vi "CreateCurveNamesvb1.vi"(8 "error in":errorcluster, 9 "NomDon":string[](array[string])=["RTêta;", "X&Y;"], 10 "IndCourbe":i64 caption="Numéro de Balayage", 11 "Experiment.lvclass In":refnum<class "Experiment.lvclass">) -> (0 "error out":errorcluster, 1 "VarPar list":string[](array[string]), 2 "Scan list":string[](array[string]), 3 "Experiment.lvclass Out":refnum<class "Experiment.lvclass">, 4 "ScanTableSize":i32[](array[numeric]))   [LabVIEW 2012]
doc: "Ce Vi créer la ligne d'entête du fichier texte de sauvegarde à partir du nombre de courbe voulu."
uses:
  DevicesClass/BaseDevice/BaseDevice.lvclass
  Calculations Class/Calculations.lvclass
  Experiment.lvclass
panel:
  out "DataQIndex":cluster{"Tableau":i32[]}[](array[cluster])
  out "CalcQIndex":cluster{"Tableau":i32[]}[](array[cluster])
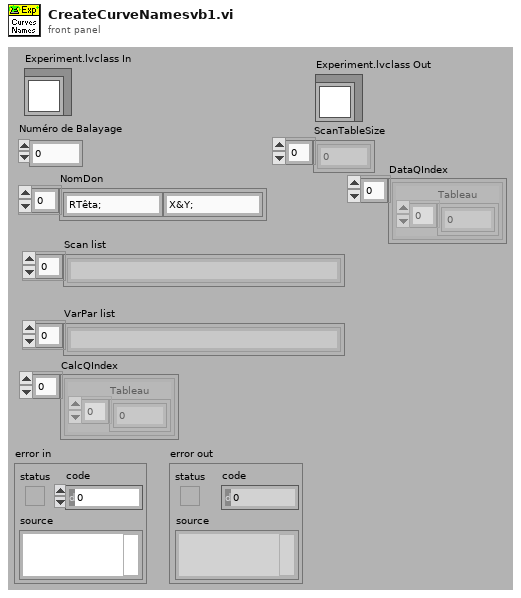
[diagram p1: front panel]
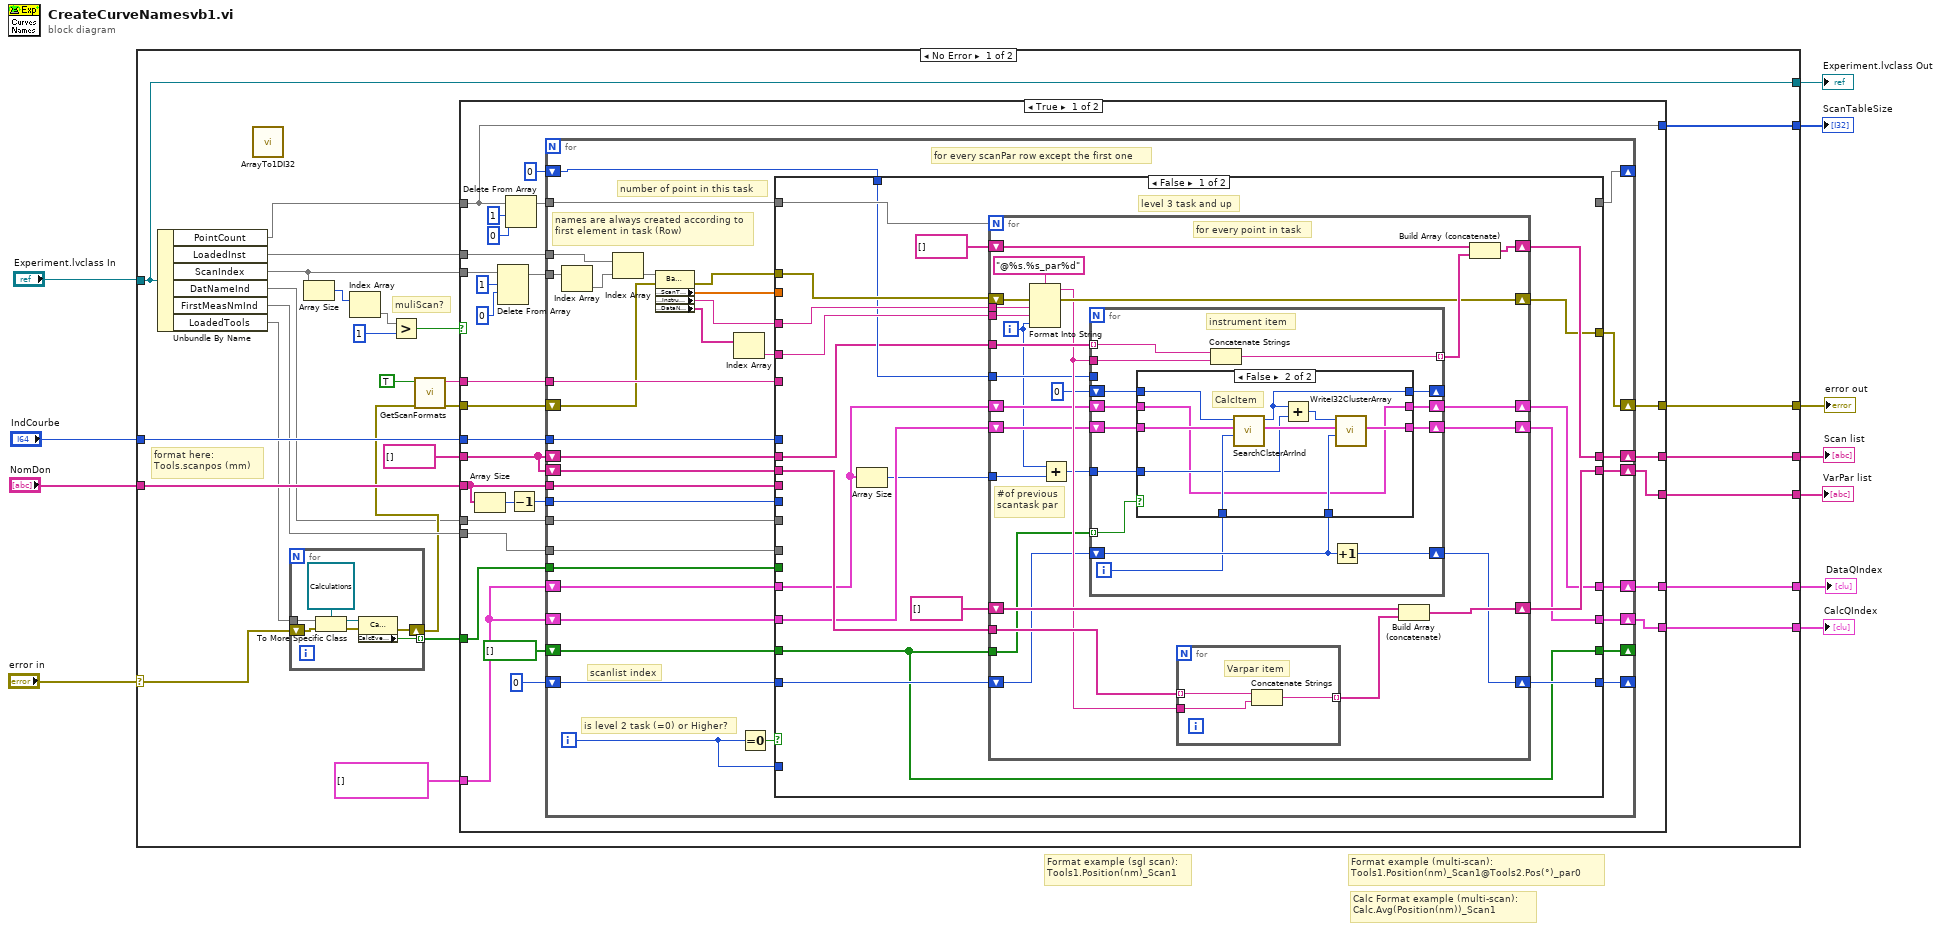
[diagram p0: block diagram]
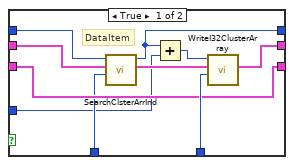
[diagram p2: hidden frame]
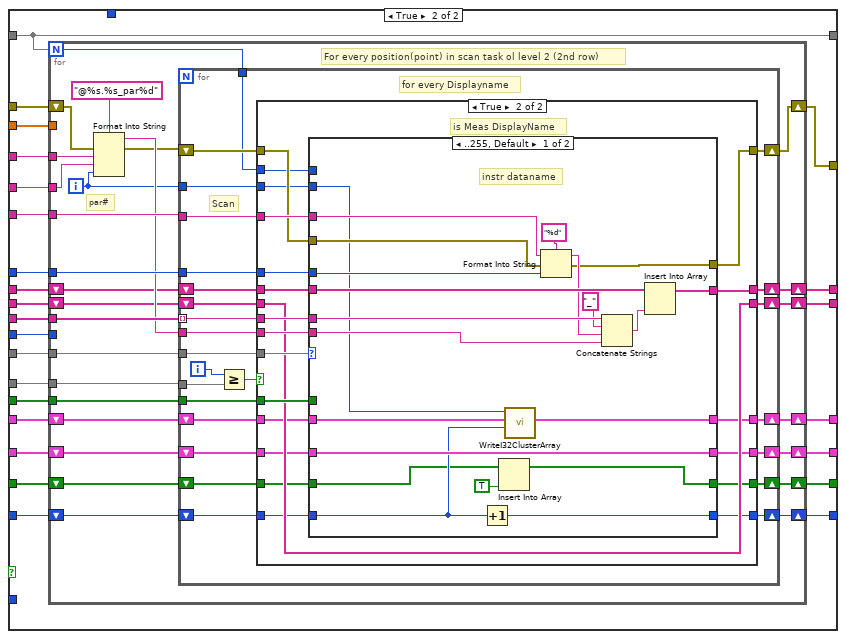
[diagram p3: hidden frame]
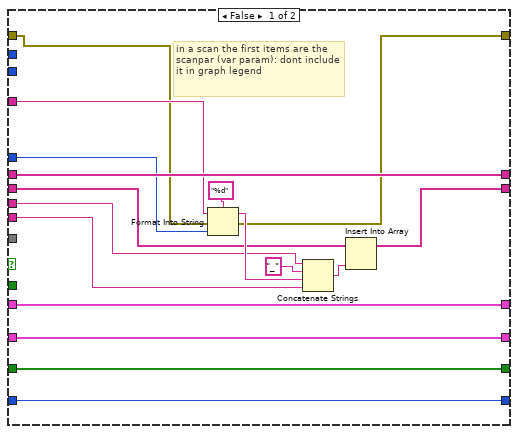
[diagram p4: hidden frame]
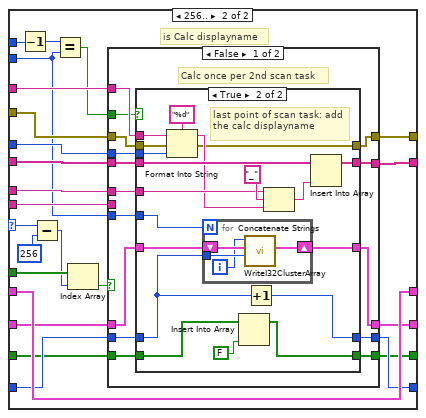
[diagram p5: hidden frame]
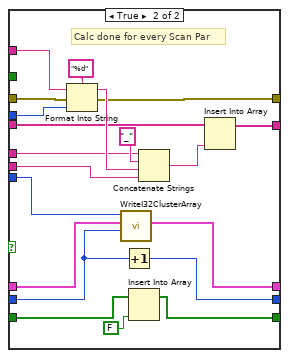
[diagram p7: hidden frame]
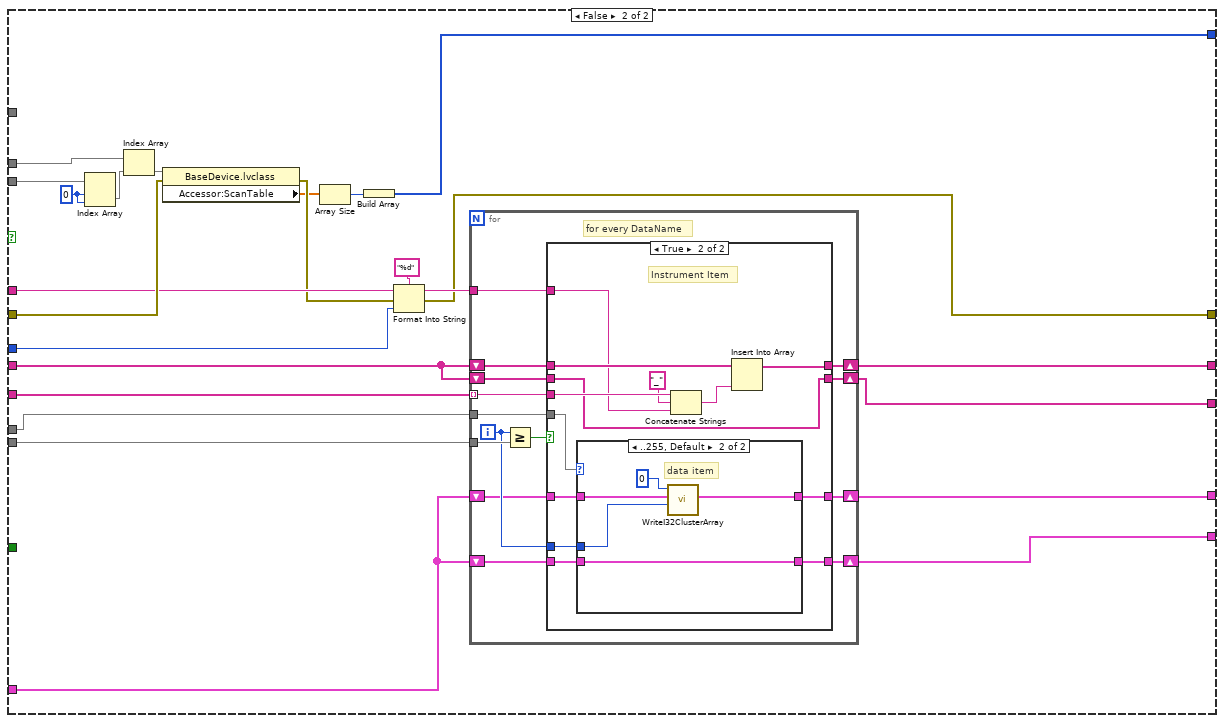
[diagram p8: hidden frame]
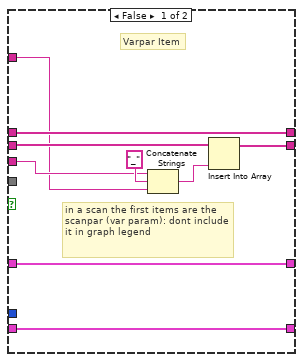
[diagram p9: hidden frame]
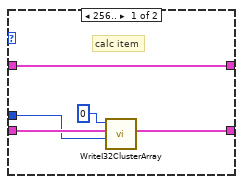
[diagram p10: hidden frame]
diagram:
  # "Calc Format example (multi-scan):\nCalc.Avg(Position(nm))_Scan1"
  # "Format example (multi-scan):\nTools1.Position(nm)_Scan1@Tools2.Pos(°)_par0"
  # "Format example (sgl scan):\nTools1.Position(nm)_Scan1"
  n1 = case shown="No Error" "error in" {
    selector: "error in" -> [w21 w486]
    tunnel: [w29 w486] -> w10
    tunnel: [w34 _] -> w9
    tunnel: "NomDon" -> [w35 _]
    tunnel: "Experiment.lvclass In" -> [w18 w485]
    tunnel: "IndCourbe" -> [w37 _]
    tunnel: [w18 w485] -> w5
    tunnel: [w26 _] -> w4
    tunnel: [w17 _] -> w3
    tunnel: [w14 _] -> w2
    tunnel: [w13 _] -> w1
    frame No Error {
      # "format here:\nTools.scanpos (mm)"
      # "muliScan?"
      n2 = Unbundle By Name(w18) -> ("PointCount"=w23, "LoadedInst"=w30, "ScanIndex"=w31, "DatNameInd"=w16, "FirstMeasNmInd"=w28, "LoadedTools"=w22)
      n3 = call <userlib>:"ArrayTo1DI32.vi"() -> ()  [unwired: 9 in, 3 out]
      n4 = for {
        tunnel: w22 -> [w42]
        shift-right: [w40] -> w20
        shift-left: w21 -> [w41]
        tunnel: [w39] -> w19 mode=indexing
        n5 = To More Specific Class(target class=refnum<class "Calculations.lvclass"> refnum ("Calculations.lvclass"), reference=w42, error in=w41) -> (specific class reference=w44:refnum<class "Calculations.lvclass">, error out=w45:errorcluster)
        n6 = property class="Calculations.lvclass"(reference=w44, error in=w45) -> (error out=w40:errorcluster, "CalcEveryScanPar"=w39:bool)  [unwired: 1 out]
      }
      n7 = Array Size(array=w31) -> (size(s)=w25:i32)
      n8 = Index Array(array=w25) -> (element=w24)  [unwired: 1 in]
      n9 = Greater?(x=w24, y=1) -> (0:w27:bool)
      n10 = call "GetScanFormats.vi"("ErrorIn(No Error)"=w20, "Scan(T)"=TRUE) -> ("sortie d'erreur"=w36:errorcluster, "Prefixe"=w38:string)  [unwired: 7 in, 1 out]
      n11 = case shown="True" w27 {
        tunnel: w38 -> [w73 w427]
        tunnel: w37 -> [w72 w428]
        tunnel: w36 -> [w71 w432]
        tunnel: w35 -> [w58 w438]
        tunnel: [w66 w437] -> w34
        tunnel: string[] [] -> [w53 w431]
        tunnel: w31 -> [w70 w435]
        tunnel: w30 -> [w69 w434]
        tunnel: [w68 w420] -> w29
        tunnel: w28 -> [w67 w436]
        tunnel: [w54 w433] -> w26
        tunnel: w23 -> [w54 _]
        tunnel: w16 -> [w59 w424]
        tunnel: w19 -> [w55 _]
        tunnel: [w52 w430] -> w17
        tunnel: cluster{"Tableau":i32[]}[] [] ("CalcQIndex") -> [w50 w422]
        tunnel: [w49 w421] -> w14
        tunnel: [w48 w423] -> w13
        frame True {
          n12 = Array Size(array=w58) -> (size(s)=w57:i32)
          n13 = Delete From Array(array=w70, length=1 ("longueur"), index (row)=0 ("indice (ligne)")) -> (array with subset deleted=w65)  [unwired: 1 in, 1 out]
          n14 = Delete From Array(array=w54, length=1 ("longueur"), index=0 ("indice")) -> (array with subset deleted=w61)  [unwired: 1 out]
          n15 = Decrement(x=w57) -> (x-1=w56:i32)
          n16 = for {
            tunnel: w73 -> [w108]
            tunnel: w72 -> [w107]
            tunnel: w58 -> [w106]
            tunnel: w65 -> [w105]
            tunnel: w69 -> [w104]
            shift-right: [w102] -> w68
            shift-left: w71 -> [w103]
            tunnel: w67 -> [w101]
            shift-right: [w98] -> w66
            shift-left: w53 -> [w97]
            tunnel: w61 -> [w78]
            tunnel: w59 -> [w90]
            tunnel: w55 -> [w89]
            tunnel: w56 -> [w88]
            shift-right: [w85] -> w52
            shift-left: w53 -> [w86]
            shift-right: [w83] -> _
            shift-left: 0 ("Numérique") -> [w84]
            shift-right: [w79] -> w49
            shift-left: w50 -> [w80]
            shift-right: [w81] -> w48
            shift-left: w50 -> [w82]
            shift-right: [w77] -> _
            shift-left: 0 ("Numérique") -> [w76]
            shift-right: [w74] -> _
            shift-left: bool[] [] -> [w75]
            i -> [w87]
            # "scanlist index"
            # "is level 2 task (=0) or Higher?"
            # "number of point in this task"
            # "names are always created according to first element in task (Row)"
            # "for every scanPar row except the first one"
            n17 = Index Array(array=w105) -> (element=w95)  [unwired: 1 in]
            n18 = Index Array(array=w104, index=w95) -> (element=w94)
            n19 = property class="BaseDevice.lvclass"(reference=w94, error in=w103) -> (error out=w96:errorcluster, "Accessor:ScanTable"=w92:dbl[], "Accessor:InstrumentName"=w99:string, "Accessor:DataNames"=w93:string[])  [unwired: 1 out]
            n20 = Index Array(array=w93) -> (element=w100:string)  [unwired: 1 in]
            n21 = Equal To 0?(x=w87) -> (x = 0?=w91:bool)
            n22 = case shown="False" w91 {
              tunnel: w108 -> [_ w216]
              tunnel: w107 -> [_ w215]
              tunnel: w106 -> [_ w214]
              tunnel: [w126 w213] -> w102
              tunnel: w101 -> [_ w212]
              tunnel: w100 -> [w124 w211]
              tunnel: w99 -> [w123 w210]
              tunnel: [w127 w209] -> w98
              tunnel: w97 -> [w113 w208]
              tunnel: w78 -> [w125 w194]
              tunnel: w96 -> [w128 w207]
              tunnel: w92 -> [_ w206]
              tunnel: w90 -> [_ w205]
              tunnel: w89 -> [_ w204]
              tunnel: w88 -> [_ w203]
              tunnel: w87 -> [_ _]
              tunnel: w86 -> [w122 w202]
              tunnel: [w121 w201] -> w85
              tunnel: w84 -> [w119 w200]
              tunnel: [w118 w199] -> w83
              tunnel: w82 -> [w112 w198]
              tunnel: [w115 w197] -> w81
              tunnel: w80 -> [w120 w196]
              tunnel: [w114 w195] -> w79
              tunnel: [_ w194] -> w77
              tunnel: w76 -> [w117 _]
              tunnel: w75 -> [w116 w193]
              tunnel: [w116 w192] -> w74
              frame False {
                # "level 3 task and up"
                n23 = Array Size(array=w112) -> (size(s)=w111:i32)
                n24 = for {
                  N: w125 -> [_]
                  tunnel: w123 -> [w154]
                  tunnel: w124 -> [w153]
                  shift-right: [w149] -> w126
                  shift-left: w128 -> [w152]
                  tunnel: w113 -> [w151]
                  shift-right: [w148] -> w127
                  shift-left: string[] [] -> [w147]
                  shift-right: [w145] -> w121
                  shift-left: string[] [] -> [w144]
                  tunnel: w122 -> [w143]
                  shift-right: [w133] -> w114
                  shift-left: w120 -> [w135]
                  shift-right: [w132] -> w118
                  shift-left: w119 -> [w140]
                  shift-right: [w134] -> w115
                  shift-left: w112 -> [w137]
                  tunnel: w117 -> [w139]
                  tunnel: w116 -> [w138]
                  tunnel: w111 -> [w131]
                  i -> [w130]
                  # "#of previous\nscantask par"
                  # "for every point in task"
                  n25 = Format Into String(format string="@%s.%s_par%d" ("chaîne de format"), error in=w152, w154, w153, w130) -> (resulting string=w141:string, error out=w149:errorcluster)  [unwired: 1 in]
                  n26 = Add(x=w130, y=w131) -> (x+y=w129:i32)
                  n27 = for {
                    tunnel: w151 -> [w168] mode=indexing
                    tunnel: [w167] -> w150 mode=indexing
                    tunnel: w141 -> [w166]
                    tunnel: w139 -> [_]
                    tunnel: w138 -> [w165] mode=indexing
                    shift-right: [w162] -> w134
                    shift-left: w137 -> [w164]
                    shift-right: [w156] -> _
                    shift-left: 0 -> [w157]
                    shift-right: [w160] -> w133
                    shift-left: w135 -> [w161]
                    shift-right: [w159] -> w132
                    shift-left: w140 -> [w163]
                    tunnel: w129 -> [w155]
                    i -> [w158]
                    # "instrument item"
                    n28 = case shown="False" w165 {
                      tunnel: w164 -> [w175 w179]
                      tunnel: w163 -> [w178 w188]
                      tunnel: [w177 w179] -> w162
                      tunnel: w161 -> [w176 w181]
                      tunnel: [w176 w180] -> w160
                      tunnel: w158 -> [w173 w186]
                      tunnel: w157 -> [w172 w185]
                      tunnel: [w171 w184] -> w156
                      tunnel: w155 -> [w170 w183]
                      frame True {
                        # "DataItem"
                        n29 = call "SearchClsterArrInd.vi"("SearchData"=w173, "array"=w175, "ClusterInd"=w172) -> ("output array"=w174:cluster{"Tableau":i32[]}[], "ClusterInd Out"=w171:i32)  [unwired: 6 in, 1 out]
                        n30 = Add(x=w171, y=w170) -> (x+y=w169:i32)
                        n31 = call <userlib>:"WriteI32ClusterArray.vi"("Data"=w178, "array"=w174, "ClusterInd"=w169) -> ("output array"=w177:cluster{"Tableau":i32[]}[])  [unwired: 7 in, 1 out]
                      }
                      frame False {
                        # "CalcItem"
                        n32 = call "SearchClsterArrInd.vi"("SearchData"=w186, "array"=w181, "ClusterInd"=w185) -> ("output array"=w187:cluster{"Tableau":i32[]}[], "ClusterInd Out"=w184:i32)  [unwired: 6 in, 1 out]
                        n33 = Add(x=w184, y=w183) -> (x+y=w182:i32)
                        n34 = call <userlib>:"WriteI32ClusterArray.vi"("Data"=w188, "array"=w187, "ClusterInd"=w182) -> ("output array"=w180:cluster{"Tableau":i32[]}[])  [unwired: 7 in, 1 out]
                      }
                    }
                    n35 = Concatenate Strings(w168, w166) -> (w167:string)
                    n36 = Increment(x=w163) -> (x+1=w159:i32)
                  }
                  n37 = for {
                    tunnel: w143 -> [w191] mode=indexing
                    tunnel: [w190] -> w146 mode=indexing
                    tunnel: w141 -> [w189]
                    # "Varpar item"
                    n38 = Concatenate Strings(w191, w189) -> (w190:string)
                  }
                  n39 = Build Array (concatenate)(w144, w146) -> (w145:string[])
                  n40 = Build Array (concatenate)(w147, w150) -> (w148:string[])
                }
              }
              frame True {
                n41 = for {
                  N: w194 -> [w230]
                  tunnel: w216 -> [w243]
                  tunnel: w215 -> [w242]
                  tunnel: w214 -> [w241]
                  shift-right: [w227] -> w213
                  shift-left: w207 -> [w239]
                  tunnel: w212 -> [w240]
                  tunnel: w211 -> [w238]
                  tunnel: w210 -> [w237]
                  shift-right: [w228] -> w209
                  shift-left: w208 -> [w235]
                  tunnel: w206 -> [_]
                  tunnel: w205 -> [w232]
                  tunnel: w204 -> [w231]
                  tunnel: w203 -> [_]
                  shift-right: [w225] -> w201
                  shift-left: w202 -> [w226]
                  shift-right: [w223] -> w199
                  shift-left: w200 -> [w224]
                  shift-right: [w221] -> w197
                  shift-left: w198 -> [w222]
                  shift-right: [w219] -> w195
                  shift-left: w196 -> [w220]
                  shift-right: [w217] -> w192
                  shift-left: w193 -> [w218]
                  i -> [w229]
                  # "par#"
                  # "For every position(point) in scan task ol level 2 (2nd row)"
                  n42 = Format Into String(format string="@%s.%s_par%d" ("chaîne de format"), error in=w239, w237, w238, w229) -> (resulting string=w236:string, error out=w234:errorcluster)  [unwired: 1 in]
                  n43 = for {
                    tunnel: w243 -> [w263]
                    tunnel: w241 -> [w266] mode=indexing
                    shift-right: [w267] -> w228
                    shift-left: w235 -> [w268]
                    tunnel: w242 -> [w264]
                    shift-right: [w254] -> w227
                    shift-left: w234 -> [w262]
                    tunnel: w240 -> [w261]
                    tunnel: w236 -> [w260]
                    tunnel: w232 -> [w259]
                    tunnel: w231 -> [w258]
                    tunnel: w230 -> [w256]
                    tunnel: w229 -> [w255]
                    shift-right: [w252] -> w225
                    shift-left: w226 -> [w253]
                    shift-right: [w250] -> w223
                    shift-left: w224 -> [w251]
                    shift-right: [w248] -> w221
                    shift-left: w222 -> [w249]
                    shift-right: [w246] -> w219
                    shift-left: w220 -> [w247]
                    shift-right: [w245] -> w217
                    shift-left: w218 -> [w244]
                    i -> [w257]
                    # "Scan"
                    # "for every Displayname"
                    n44 = Greater Or Equal?(x=w257, y=w261) -> (x >= y?=w265:bool)
                    n45 = case shown="True" w265 {
                      tunnel: w268 -> [w285 w306]
                      tunnel: [w285 w305] -> w267
                      tunnel: w266 -> [w279 w304]
                      tunnel: w264 -> [w273 w300]
                      tunnel: w263 -> [w280 w303]
                      tunnel: w262 -> [w277 w302]
                      tunnel: w260 -> [w278 w301]
                      tunnel: w259 -> [_ w298]
                      tunnel: w258 -> [_ w299]
                      tunnel: w256 -> [_ w297]
                      tunnel: w255 -> [_ w296]
                      tunnel: [w276 w295] -> w254
                      tunnel: w253 -> [w275 w294]
                      tunnel: [w274 w294] -> w252
                      tunnel: w251 -> [w272 w289]
                      tunnel: [w272 w288] -> w250
                      tunnel: w249 -> [w271 w293]
                      tunnel: [w271 w292] -> w248
                      tunnel: w247 -> [w270 w291]
                      tunnel: [w270 w290] -> w246
                      tunnel: [w269 w286] -> w245
                      tunnel: w244 -> [w269 w287]
                      frame False {
                        # "in a scan the first items are the scanpar (var param): dont include it in graph legend"
                        n46 = Format Into String(format string="%d" ("chaîne de format"), initial string=w280, error in=w277, w273) -> (resulting string=w283:string, error out=w276:errorcluster)
                        n47 = Concatenate Strings(w279, "_" ("chaîne"), w283, w278) -> (w284:string)
                        n48 = Insert Into Array(array=w275, new element=w284) -> (w274:string[])  [unwired: 1 in]
                      }
                      frame True {
                        # "is Meas DisplayName"
                        n49 = case shown="..255, Default" w298 {
                          selector: w298 -> [_ w342]
                          tunnel: w306 -> [w327 w348]
                          tunnel: [w326 w346] -> w305
                          tunnel: w304 -> [w325 w349]
                          tunnel: w303 -> [w324 w351]
                          tunnel: w302 -> [w323 w337]
                          tunnel: w301 -> [w319 w347]
                          tunnel: w300 -> [w318 w350]
                          tunnel: w299 -> [_ w345]
                          tunnel: w297 -> [_ w341]
                          tunnel: w296 -> [w313 w333]
                          tunnel: [w316 w338] -> w295
                          tunnel: w293 -> [w315 w335]
                          tunnel: w289 -> [w311 w330]
                          tunnel: [w314 w335] -> w292
                          tunnel: w291 -> [w312 w334]
                          tunnel: [w312 w332] -> w290
                          tunnel: [w310 w331] -> w288
                          tunnel: w287 -> [w309 w329]
                          tunnel: [w307 w328] -> w286
                          frame ..255, Default {
                            # "instr dataname"
                            n50 = Increment(x=w311) -> (x+1=w310:i32)
                            n51 = Insert Into Array(array=w309, new element=TRUE ("new element/subarray")) -> (w307:bool[])  [unwired: 1 in]
                            n52 = call <userlib>:"WriteI32ClusterArray.vi"("Data"=w311, "array"=w315, "ClusterInd"=w313) -> ("output array"=w314:cluster{"Tableau":i32[]}[])  [unwired: 7 in, 1 out]
                            n53 = Format Into String(format string="%d" ("chaîne de format"), initial string=w324, error in=w323, w318) -> (resulting string=w321:string, error out=w316:errorcluster)
                            n54 = Concatenate Strings(w325, "_" ("chaîne"), w321, w319) -> (w322:string)
                            n55 = Insert Into Array(array=w327, new element=w322) -> (w326:string[])  [unwired: 1 in]
                          }
                          frame 256.. {
                            # "is Calc displayname"
                            n56 = Decrement(x=w341) -> (x-1=w340:i32)
                            n57 = Subtract(x=w342, y=256) -> (x-y=w344:i32)
                            n58 = Equal?(x=w340, y=w333) -> (x = y?=w339:bool)
                            n59 = Index Array(array=w345, index=w344) -> (element=w336:bool)
                            n60 = case shown="False" w336 {
                              tunnel: w351 -> [w362 w410]
                              tunnel: w350 -> [w366 w409]
                              tunnel: w349 -> [w364 w408]
                              tunnel: w348 -> [w365 w407]
                              tunnel: w347 -> [_ w405]
                              tunnel: [w363 w406] -> w346
                              tunnel: w339 -> [w361 _]
                              tunnel: [w360 w404] -> w338
                              tunnel: w337 -> [w359 w403]
                              tunnel: w334 -> [w358 w400]
                              tunnel: w330 -> [w355 w399]
                              tunnel: w333 -> [w356 w402]
                              tunnel: [w357 w401] -> w332
                              tunnel: [w354 w398] -> w331
                              tunnel: w329 -> [w353 w397]
                              tunnel: [w352 w395] -> w328
                              frame False {
                                # "Calc once per 2nd scan task"
                                n61 = case shown="True" w361 {
                                tunnel: w362 -> [_ w389]
                                tunnel: w366 -> [_ w388]
                                tunnel: w365 -> [w371 w385]
                                tunnel: w364 -> [_ w384]
                                tunnel: [w371 w382] -> w363
                                tunnel: [w370 w381] -> w360
                                tunnel: w359 -> [w370 w380]
                                tunnel: w358 -> [w369 w376]
                                tunnel: [w369 w378] -> w357
                                tunnel: w356 -> [_ w379]
                                tunnel: w355 -> [w368 w377]
                                tunnel: [w368 w375] -> w354
                                tunnel: w353 -> [w367 w373]
                                tunnel: [w367 w372] -> w352
                                frame False {
                                }
                                frame True {
                                # "last point of scan task: add the calc displayname"
                                n62 = Format Into String(format string="%d" ("chaîne de format"), initial string=w389, error in=w380, w388) -> (resulting string=w383:string, error out=w381:errorcluster)
                                n63 = for {
                                N: w379 -> [_]
                                tunnel: w377 -> [w393]
                                shift-right: [w391] -> w378
                                shift-left: w376 -> [w394]
                                i -> [w392]
                                n64 = call <userlib>:"WriteI32ClusterArray.vi"("Data"=w393, "array"=w394, "ClusterInd"=w392) -> ("output array"=w391:cluster{"Tableau":i32[]}[])  [unwired: 7 in, 1 out]
                                }
                                n65 = Insert Into Array(array=w373, new element=FALSE ("new element/subarray")) -> (w372:bool[])  [unwired: 1 in]
                                n66 = Increment(x=w377) -> (x+1=w375:i32)
                                n67 = Concatenate Strings(w384, "_" ("chaîne"), w383) -> (w386:string)
                                n68 = Insert Into Array(array=w385, new element=w386) -> (w382:string[])  [unwired: 1 in]
                                }
                                }
                              }
                              frame True {
                                # "Calc done for every Scan Par"
                                n69 = Format Into String(format string="%d" ("chaîne de format"), initial string=w410, error in=w403, w409) -> (resulting string=w412:string, error out=w404:errorcluster)
                                n70 = call <userlib>:"WriteI32ClusterArray.vi"("Data"=w399, "array"=w400, "ClusterInd"=w402) -> ("output array"=w401:cluster{"Tableau":i32[]}[])  [unwired: 7 in, 1 out]
                                n71 = Increment(x=w399) -> (x+1=w398:i32)
                                n72 = Insert Into Array(array=w397, new element=FALSE ("new element/subarray")) -> (w395:bool[])  [unwired: 1 in]
                                n73 = Concatenate Strings(w408, "_" ("chaîne"), w412, w405) -> (w411:string)
                                n74 = Insert Into Array(array=w407, new element=w411) -> (w406:string[])  [unwired: 1 in]
                              }
                            }
                          }
                        }
                      }
                    }
                  }
                }
              }
            }
          }
        }
        frame False {
          w417 = 0 ("indice (ligne)")
          n75 = Index Array(array=w435, index (row)=w417, index (col)=w417) -> (element=w419)
          n76 = Index Array(array=w434, index=w419) -> (element=w418)
          n77 = property class="BaseDevice.lvclass"(reference=w418, error in=w432) -> (error out=w425:errorcluster, "Accessor:ScanTable"=w416:dbl[])  [unwired: 1 out]
          n78 = Array Size(array=w416) -> (size(s)=w415:i32)
          n79 = Build Array(w415) -> (w433:i32[])
          n80 = Format Into String(format string="%d" ("chaîne de format"), initial string=w427, error in=w425, w428) -> (resulting string=w426:string, error out=w420:errorcluster)
          n81 = for {
            tunnel: w426 -> [w448]
            tunnel: w438 -> [w450] mode=indexing
            shift-right: [w451] -> w437
            shift-left: w431 -> [w452]
            tunnel: w436 -> [w447]
            shift-right: [w445] -> w430
            shift-left: w431 -> [w446]
            tunnel: w424 -> [w444]
            shift-right: [w440] -> w423
            shift-left: w422 -> [w439]
            shift-right: [w442] -> w421
            shift-left: w422 -> [w443]
            i -> [w441]
            # "for every DataName"
            n82 = Greater Or Equal?(x=w441, y=w447) -> (x >= y?=w449:bool)
            n83 = case shown="True" w449 {
              tunnel: w452 -> [w461 w474]
              tunnel: [w461 w473] -> w451
              tunnel: w450 -> [w456 w472]
              tunnel: w448 -> [w455 w470]
              tunnel: w446 -> [w458 w471]
              tunnel: [w457 w471] -> w445
              tunnel: w444 -> [_ w467]
              tunnel: w443 -> [w454 w466]
              tunnel: [w454 w465] -> w442
              tunnel: w441 -> [_ w464]
              tunnel: [w453 w463] -> w440
              tunnel: w439 -> [w453 w462]
              frame False {
                # "in a scan the first items are the scanpar (var param): dont include it in graph legend"
                # "Varpar Item"
                n84 = Concatenate Strings(w456, "_" ("chaîne"), w455) -> (w460:string)
                n85 = Insert Into Array(array=w458, new element=w460) -> (w457:string[])  [unwired: 1 in]
              }
              frame True {
                # "Instrument Item"
                n86 = case shown="..255, Default" w467 {
                  tunnel: w466 -> [w479 w484]
                  tunnel: [w478 w484] -> w465
                  tunnel: w464 -> [w476 w480]
                  tunnel: [w475 w481] -> w463
                  tunnel: w462 -> [w475 w482]
                  frame 256.. {
                    # "calc item"
                    n87 = call <userlib>:"WriteI32ClusterArray.vi"("Data"=w476, "array"=w479, "ClusterInd"=0) -> ("output array"=w478:cluster{"Tableau":i32[]}[])  [unwired: 7 in, 1 out]
                  }
                  frame ..255, Default {
                    # "data item"
                    n88 = call <userlib>:"WriteI32ClusterArray.vi"("Data"=w480, "array"=w482, "ClusterInd"=0) -> ("output array"=w481:cluster{"Tableau":i32[]}[])  [unwired: 7 in, 1 out]
                  }
                }
                n89 = Concatenate Strings(w472, "_" ("chaîne"), w470) -> (w469:string)
                n90 = Insert Into Array(array=w474, new element=w469) -> (w473:string[])  [unwired: 1 in]
              }
            }
          }
        }
      }
    }
    frame Error {
    }
  }
  "error out" <- w10
  "Scan list" <- w9
  "Experiment.lvclass Out" <- w5
  "ScanTableSize" <- w4
  "VarPar list" <- w3
  "CalcQIndex" <- w2
  "DataQIndex" <- w1
